vi "Thermometer (Demo).vi"(2 "error in (no error)":errorcluster, 3 "Temp Scale":bool) -> (0 "error out":errorcluster, 1 "Temperature":dbl(slide) scale=0.0..100.0 scale format="%.1f")   [LabVIEW 2016]
doc: "This VI simulates measuring a temperature using the temperature sensor on the DAQ Signal Accessory.\n\nIf you have a DAQ board or a DAQ Signal Accessory, then use the Thermometer VI instead."
panel:
  # "deg C\n\ndeg F"
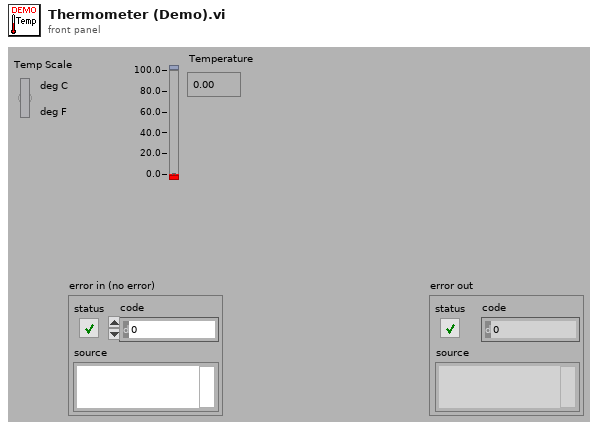
[diagram p1: front panel]
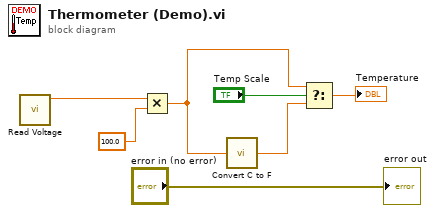
[diagram p0: block diagram]
diagram:
  n1 = call "Read Voltage.vi"() -> ("voltage"=w2:dbl)  [unwired: 6 in, 1 out]
  n2 = Multiply(x=w2, y=100.0) -> (x*y=w3:dbl)
  n3 = call "Convert C to F.vi"("deg C"=w3) -> ("deg F"=w6:dbl)
  n4 = Select(t=w3, s="Temp Scale", f=w6) -> (s? t:f=→"Temperature":dbl)
  "error out" <- "error in (no error)"
